vi "RT_TVA_DATA_vPXI.vi"(11 "TVA data":u8[](array[numeric])) -> (0 "Roll Rate/angle":dbl[](array[numeric]), 2 "Yaw Angle":dbl(knob) scale=-3.0..3.0, 3 "Pitch Angle":dbl(knob) scale=-3.0..3.0, 4 "CRC Check over Byte #10 to byte #29":bool, 5 "Control Variables (extra variables)":dbl[](array[numeric]), 6 "CRC Check over Byte #2 to Byte #7":bool)   [LabVIEW 2017]
panel:
  out "output array":u8[](array[numeric]) format="%x"
  out "CRC data":u16 format="%x"
  out "CRC data comp":u16 format="%x"
  out "CRC addr":u16 format="%x"
  out "CRC addr comp":u16 format="%x"
  out "Roll DMARS":dbl
  out "commando3":dbl
  out "Yaw DMARS":dbl
  out "Pitch DMARS":dbl
  out "Roll Angle":dbl
  out "Roll Rate":dbl
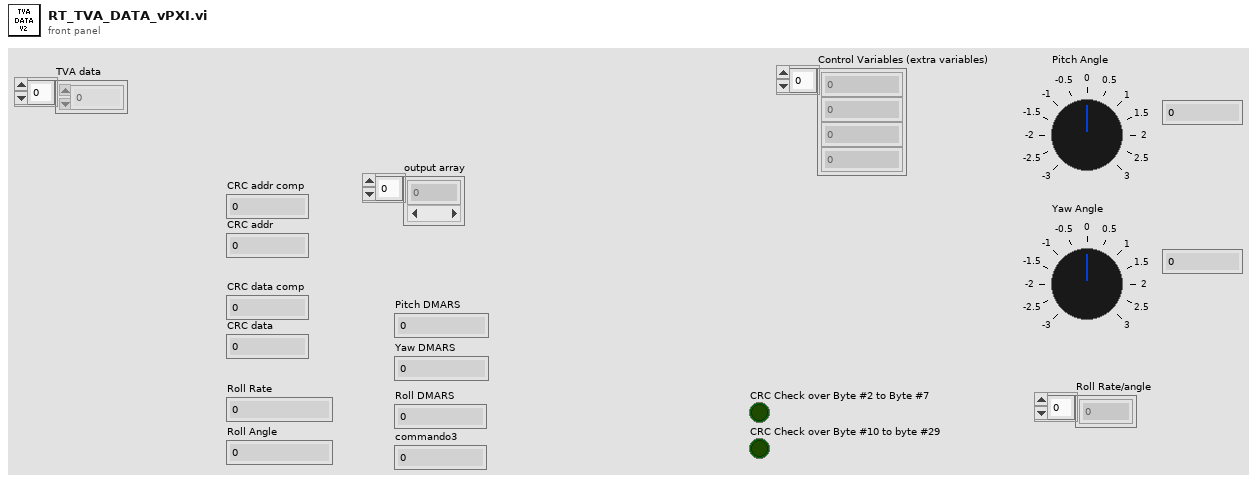
[diagram p1: front panel]
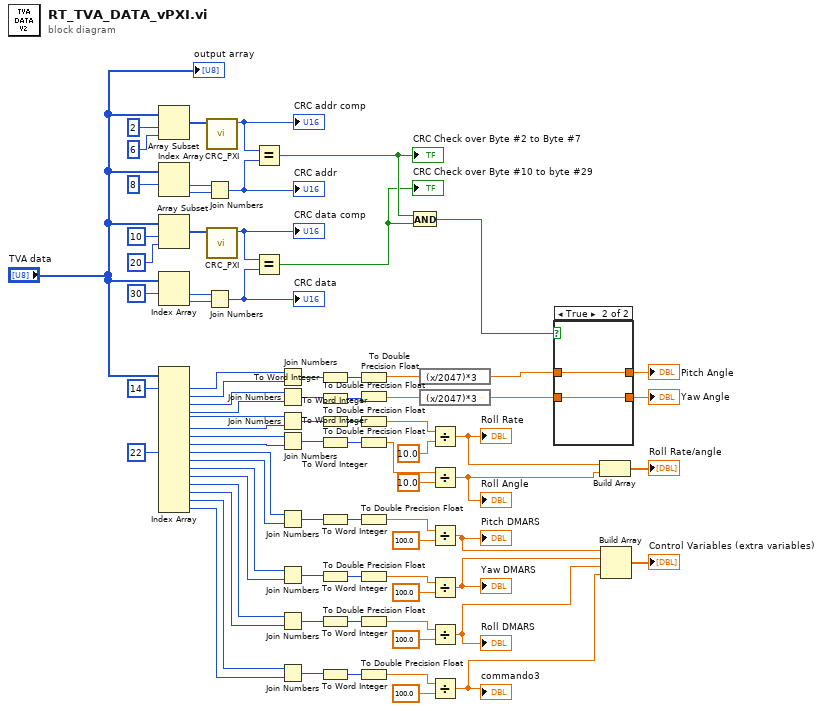
[diagram p0: block diagram]
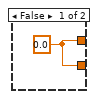
[diagram p2: hidden frame]
diagram:
  n1 = Array Subset(array="TVA data", index=2, length=6) -> (w21:u8[])
  n2 = Index Array(array="TVA data", index #1=8 ("index")) -> (element #1=w17:u8, element #2=w18:u8)  [unwired: 1 in]
  n3 = Array Subset(array="TVA data", index=10, length=20) -> (w11:u8[])
  n4 = Index Array(array="TVA data", index #1=30 ("index")) -> (element #1=w14:u8, element #2=w13:u8)  [unwired: 1 in]
  n5 = Index Array(array="TVA data", index #1=14 ("index"), index #9=22 ("index")) -> (element #1=w75:u8, element #2=w76:u8, element #3=w77:u8, element #4=w78:u8, element #5=w68:u8, element #6=w67:u8, element #7=w66:u8, element #8=w65:u8, element #9=w30:u8, element #10=w31:u8, element #11=w29:u8, element #12=w28:u8, element #13=w43:u8, element #14=w42:u8, element #15=w41:u8, element #16=w40:u8)  [unwired: 14 in]
  n6 = Join Numbers(hi=w17, lo=w18) -> ((hi.lo)=w16:u16)
  "CRC addr" <- w16
  n7 = Join Numbers(hi=w14, lo=w13) -> ((hi.lo)=w2:u16)
  "CRC data" <- w2
  n8 = call "CRC_PXI.vi"("Array"=w21) -> ("CRC"=w20:u16)  [unwired: 10 in]
  "CRC addr comp" <- w20
  n9 = call "CRC_PXI.vi"("Array"=w11) -> ("CRC"=w3:u16)  [unwired: 10 in]
  "CRC data comp" <- w3
  n10 = Equal?(x=w20, y=w16) -> (x = y?=w15:bool)
  "CRC Check over Byte #2 to Byte #7" <- w15
  n11 = Equal?(x=w3, y=w2) -> (x = y?=w8:bool)
  "CRC Check over Byte #10 to byte #29" <- w8
  n12 = Join Numbers(hi=w75, lo=w76) -> ((hi.lo)=w60:u16)
  n13 = Join Numbers(hi=w77, lo=w78) -> ((hi.lo)=w58:u16)
  n14 = Join Numbers(hi=w68, lo=w67) -> ((hi.lo)=w56:u16)
  n15 = Join Numbers(hi=w66, lo=w65) -> ((hi.lo)=w55:u16)
  n16 = Join Numbers(hi=w30, lo=w31) -> ((hi.lo)=w48:u16)
  n17 = Join Numbers(hi=w29, lo=w28) -> ((hi.lo)=w49:u16)
  n18 = Join Numbers(hi=w43, lo=w42) -> ((hi.lo)=w47:u16)
  n19 = Join Numbers(hi=w41, lo=w40) -> ((hi.lo)=w46:u16)
  n20 = To Word Integer(number=w60) -> (16bit integer=w59:i16)
  n21 = To Word Integer(number=w58) -> (16bit integer=w57:i16)
  n22 = To Word Integer(number=w56) -> (16bit integer=w53:i16)
  n23 = To Word Integer(number=w55) -> (16bit integer=w54:i16)
  n24 = To Word Integer(number=w48) -> (16bit integer=w51:i16)
  n25 = To Word Integer(number=w49) -> (16bit integer=w50:i16)
  n26 = To Word Integer(number=w47) -> (16bit integer=w44:i16)
  n27 = To Word Integer(number=w46) -> (16bit integer=w45:i16)
  n28 = To Double Precision Float(number=w59) -> (double precision float=w80:dbl)
  n29 = To Double Precision Float(number=w57) -> (double precision float=w79:dbl)
  n30 = To Double Precision Float(number=w53) -> (double precision float=w61:dbl)
  n31 = To Double Precision Float(number=w54) -> (double precision float=w62:dbl)
  n32 = To Double Precision Float(number=w51) -> (double precision float=w38:dbl)
  n33 = To Double Precision Float(number=w50) -> (double precision float=w34:dbl)
  n34 = To Double Precision Float(number=w44) -> (double precision float=w33:dbl)
  n35 = To Double Precision Float(number=w45) -> (double precision float=w32:dbl)
  n36 = And(x=w15, y=w8) -> (x .and. y?=w73:bool)
  n37 = expression code="(x/2047)*3"(w80) -> (w70:dbl)
  n38 = expression code="(x/2047)*3"(w79) -> (w69:dbl)
  n39 = Divide(x=w61, y=10.0) -> (x/y=w6:dbl)
  "Roll Rate" <- w6
  n40 = Divide(x=w62, y=10.0) -> (x/y=w5:dbl)
  "Roll Angle" <- w5
  n41 = Divide(x=w38, y=100.0) -> (x/y=w27:dbl)
  "Pitch DMARS" <- w27
  n42 = Divide(x=w34, y=100.0) -> (x/y=w26:dbl)
  "Yaw DMARS" <- w26
  n43 = Divide(x=w33, y=100.0) -> (x/y=w25:dbl)
  "Roll DMARS" <- w25
  n44 = Divide(x=w32, y=100.0) -> (x/y=w7:dbl)
  "commando3" <- w7
  n45 = case shown="True" w73 {
    tunnel: [w81 w83] -> w72
    tunnel: [w81 w82] -> w71
    tunnel: w70 -> [_ w83]
    tunnel: w69 -> [_ w82]
    frame False {
      w81 = 0.0
    }
    frame True {
    }
  }
  "Yaw Angle" <- w71
  "Pitch Angle" <- w72
  n46 = Build Array(w6, w5) -> (→"Roll Rate/angle":dbl[])
  n47 = Build Array(w27, w26, w25, w7) -> (→"Control Variables (extra variables)":dbl[])
  "output array" <- "TVA data"
